vi "Get Grid Target Cell Info.vi"(1 "Simulation Object in":refnum<class "SimulationObject.lvclass">, 2 "Collision Grid in":refnum<class "CollisionGrid.lvclass">) -> (0 "info":T1)   [LabVIEW 2022 SP3, in "CollisionGrid.lvclass"]
uses:
  CollisionGrid.lvclass
  SimulationObject/SimulationObject.lvclass
  Circle Collider/Circle Collider.lvclass
  SimulationObject/SimulationObject.lvclass/SimulationObject.ctl
  CollisionGrid.lvclass/CollisionGrid.ctl
  Rect Collider/Rect Collider.lvclass
  Rect Collider/Rect Collider.lvclass/Rect Collider.ctl
  Rect Collider/Read Width.vi
  Rect Collider/Read Height.vi
  Collider/Collider.lvclass
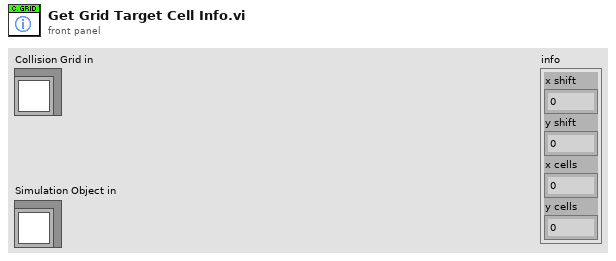
[diagram p1: front panel]
types:
  T1 = cluster{"x shift":i16, "y shift":i16, "x cells":i16, "y cells":i16}
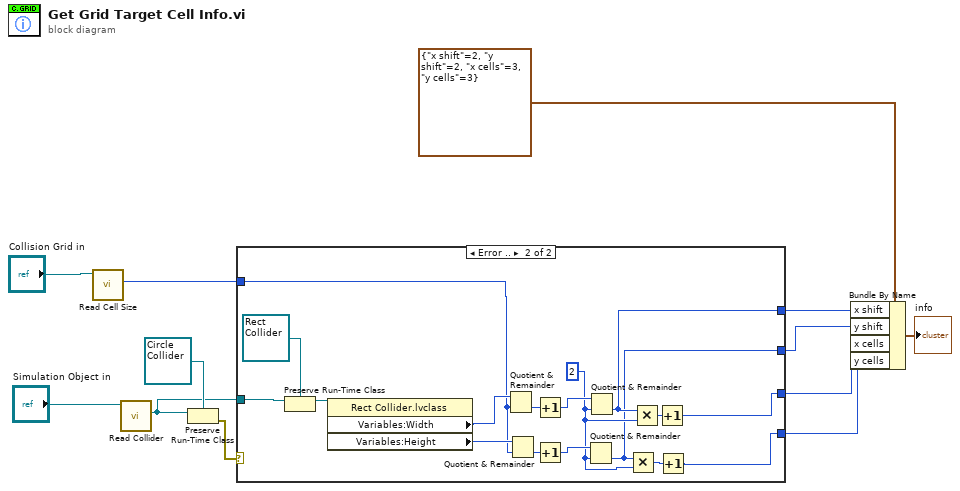
[diagram p0: block diagram]
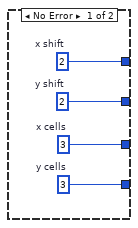
[diagram p2: hidden frame]
diagram:
  n1 = call "Read Cell Size.vi"("CollisionGrid in"="Collision Grid in") -> ("Cell Size"=w7:i16)  [unwired: 8 in, 2 out]
  n2 = call "Read Collider.vi"("SimulationObject in"="Simulation Object in") -> ("Collider out"=w10:refnum<class "Collider.lvclass">)  [unwired: 8 in, 2 out]
  n3 = Preserve Run-Time Class(object in=w10, 2:refnum<class "Circle Collider.lvclass"> refnum ("Circle Collider.lvclass")) -> (error out=w11:errorcluster)  [unwired: 1 in, 1 out]
  n4 = case shown="Error .." w11 {
    tunnel: w10 -> [_ w33]
    tunnel: [w16 w20] -> w6
    tunnel: [w15 w18] -> w5
    tunnel: [w14 w22] -> w4
    tunnel: [w13 w21] -> w3
    tunnel: w7 -> [_ w17]
    frame No Error {
      w13 = i16 3  # y cells
      w14 = i16 3  # x cells
      w15 = i16 2  # y shift
      w16 = i16 2  # x shift
    }
    frame Error {
      w19 = i16 2 ("y")
      n5 = Preserve Run-Time Class(object in=w33, 2:refnum<class "Rect Collider.lvclass"> refnum ("Rect Collider.lvclass")) -> (object out=w31:refnum<class "Rect Collider.lvclass">)  [unwired: 1 in, 1 out]
      n6 = property class="Rect Collider.lvclass"(reference=w31) -> ("Variables:Width"=w30:i16, "Variables:Height"=w29:i16)  [unwired: 1 in, 2 out]
      n7 = Quotient & Remainder(x=w30, y=w17) -> (floor(x/y)=w28:i16)  [unwired: 1 out]
      n8 = Quotient & Remainder(x=w29, y=w17) -> (floor(x/y)=w27:i16)  [unwired: 1 out]
      n9 = Increment(x=w28) -> (x+1=w26:i16)
      n10 = Increment(x=w27) -> (x+1=w25:i16)
      n11 = Quotient & Remainder(x=w25, y=w19) -> (floor(x/y)=w18:i16)  [unwired: 1 out]
      n12 = Quotient & Remainder(x=w26, y=w19) -> (floor(x/y)=w20:i16)  [unwired: 1 out]
      n13 = Multiply(x=w18, y=w19) -> (x*y=w23:i16)
      n14 = Multiply(x=w20, y=w19) -> (x*y=w24:i16)
      n15 = Increment(x=w24) -> (x+1=w22:i16)
      n16 = Increment(x=w23) -> (x+1=w21:i16)
    }
  }
  n17 = Bundle By Name(cluster=T1 {"x shift"=2, "y shift"=2, "x cells"=3, "y cells"=3}, "x shift"=w6, "y shift"=w5, "x cells"=w4, "y cells"=w3) -> (→"info":T1)
